vi "Tcp ip main.vi"() -> ()   [LabVIEW 2017]
uses:
  tcp ip server.lvclass
  Q Driver/Controls/IPC-TCP IP-Q driver-Q Options.ctl
  Q Driver/Controls/IPC-TCP IP-Q driver-En Q Element.ctl
panel:
  in  "error in (no error)":errorcluster
  out "error out":errorcluster
  out "Write Data":dbl
  out "Read Data":dbl
  in  "stop":bool
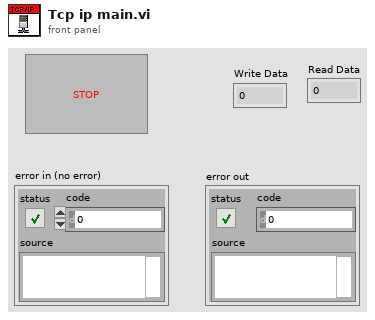
[diagram p1: front panel]
types:
  T1 = typedef "IPC-TCP IP-Q driver-Q Options.ctl" = enum16{"En Q N", "De Q", "Init", "En Q N Stack", "Flush", "Close"}
  T2 = typedef "IPC-TCP IP-Q driver-En Q Element.ctl" = cluster{"State":string, "Data":variant}
  T3 = enum16{"Init", "send", "receive", "Read Received Data", "Write Send Data"}
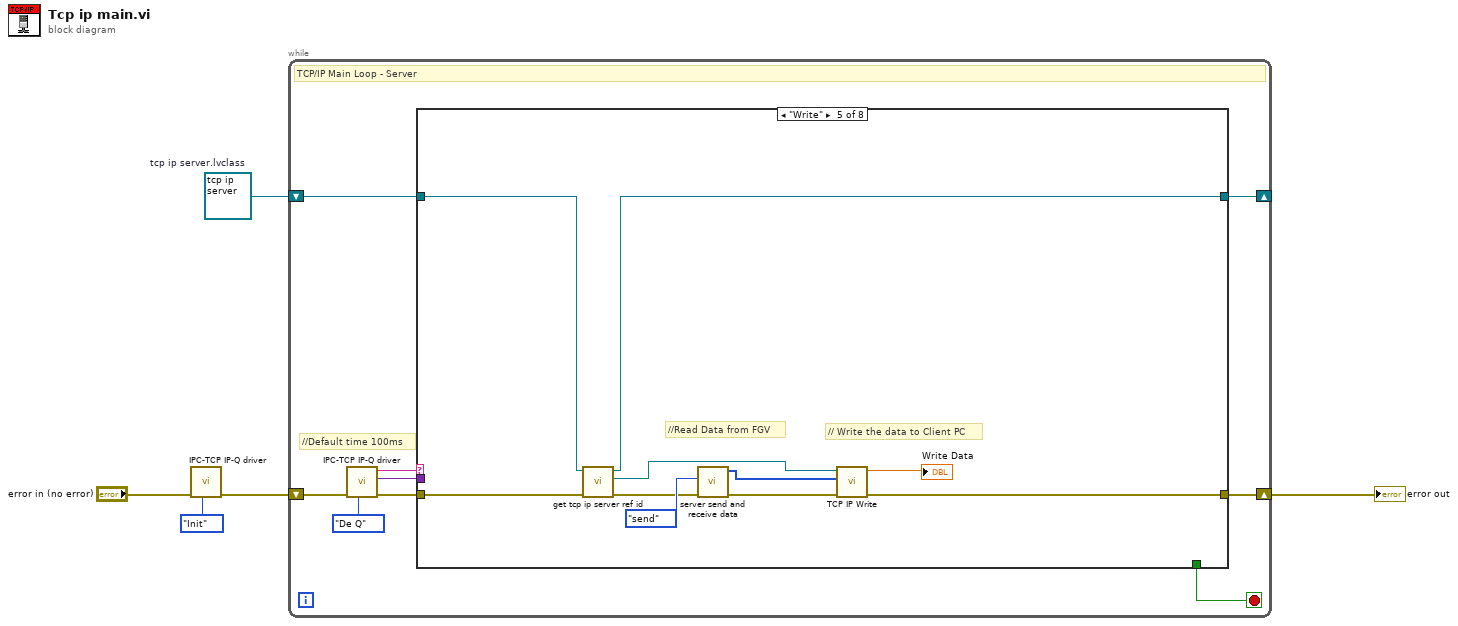
[diagram p0: block diagram]
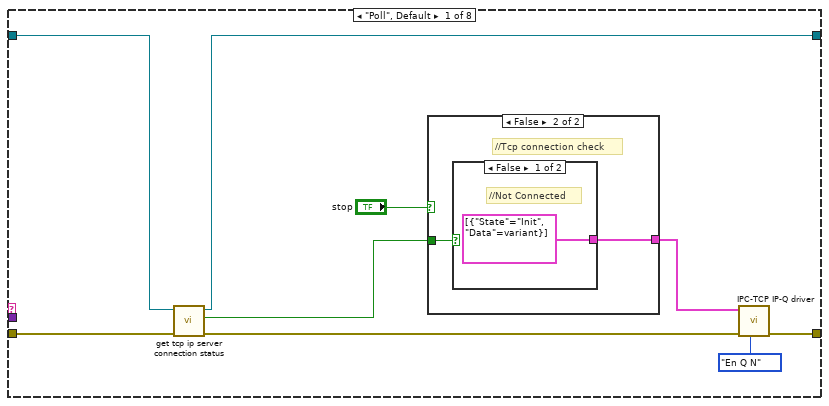
[diagram p2: hidden frame]
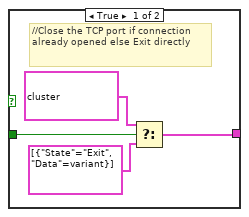
[diagram p3: hidden frame]
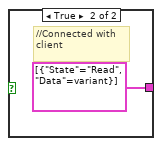
[diagram p4: hidden frame]
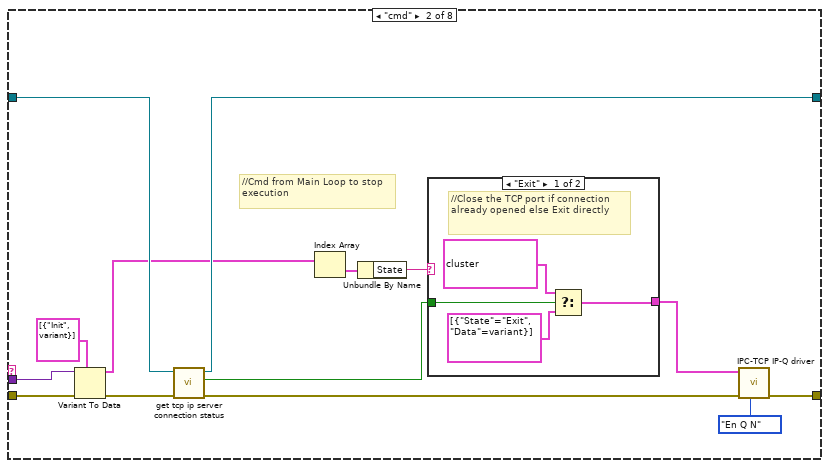
[diagram p5: hidden frame]
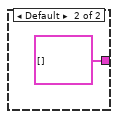
[diagram p6: hidden frame]
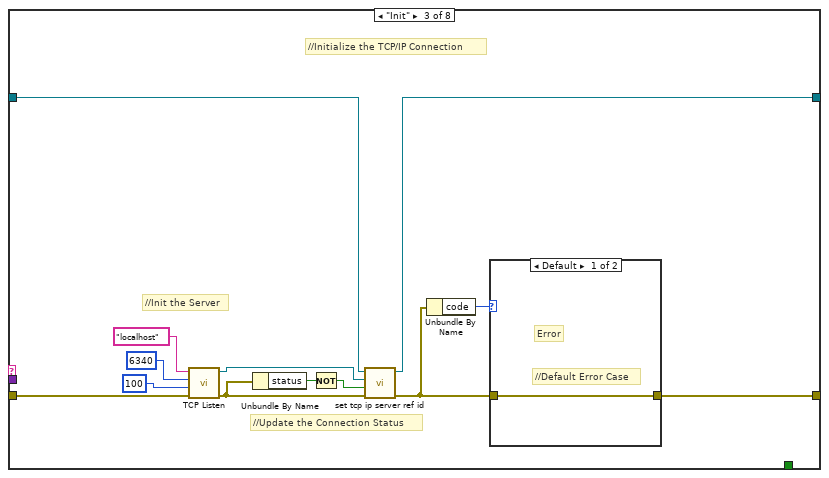
[diagram p7: hidden frame]
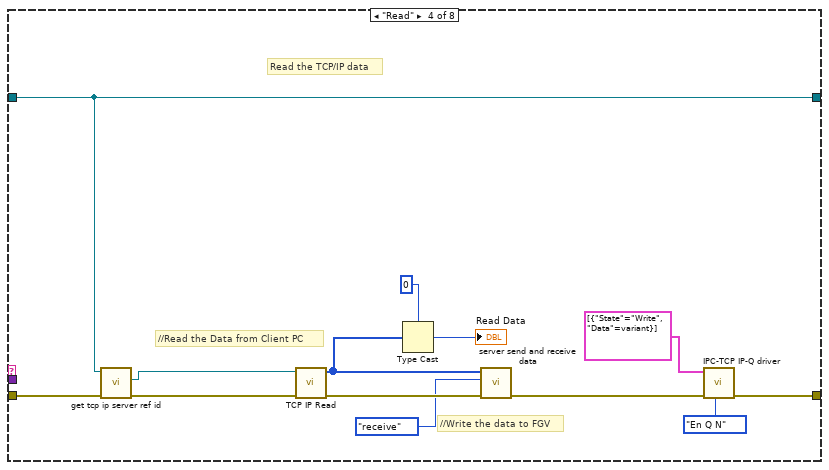
[diagram p9: hidden frame]
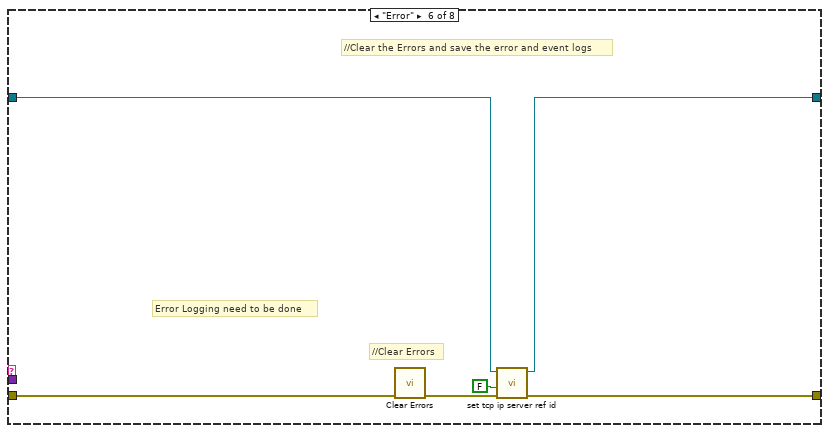
[diagram p10: hidden frame]
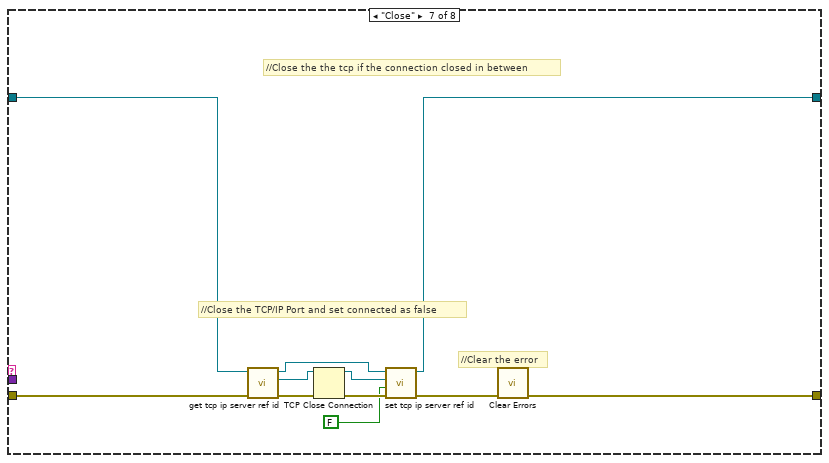
[diagram p11: hidden frame]
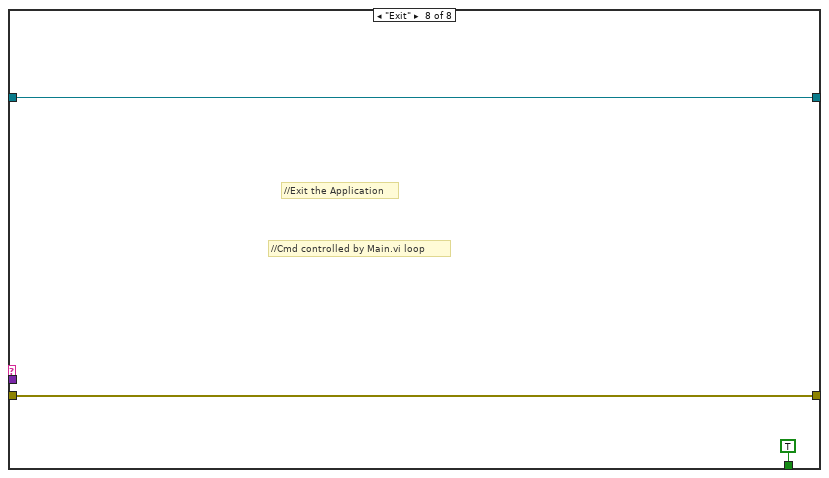
[diagram p12: hidden frame]
diagram:
  w5 = refnum<class "tcp ip server.lvclass"> refnum  # tcp ip server.lvclass
  n1 = call "IPC-TCP IP-Q driver.vi"("Q Options"=IPC-TCP_IP-Q_driver-Q_Options."Init", "error in (no error)"="error in (no error)") -> ("error out"=w4:errorcluster)  [unwired: 7 in, 2 out]
  n2 = while {
    shift-right: [w13] -> _
    shift-left: w5 -> [w14]
    shift-right: [w12] -> w2
    shift-left: w4 -> [w9]
    stop <- w11 stop-if-true
    # "//Default time 100ms"
    # "TCP/IP Main Loop - Server"
    n3 = call "IPC-TCP IP-Q driver.vi"("Q Options"=IPC-TCP_IP-Q_driver-Q_Options."De Q", "error in (no error)"=w9) -> ("error out"=w8:errorcluster, "Data"=w6:variant, "State"=w7:string)  [unwired: 7 in]
    n4 = case shown="\"Write\"" w7 {
      tunnel: w14 -> [w23 w45 w61 w75 w82 w90 w102 w106]
      tunnel: [w22 w44 w60 w75 w78 w89 w97 w106] -> w13
      tunnel: [w19 w41 w54 w67 w80 w88 w94 w105] -> w12
      tunnel: w8 -> [w16 w35 w59 w77 w86 w93 w103 w105]
      tunnel: [_ _ _ _ _ _ _ TRUE ("stop")] -> w11
      tunnel: w6 -> [_ w39 _ _ _ _ _ _]
      frame "Poll", Default {
        n5 = call-dynamic "get tcp ip server connection status.vi"("error in (no error)"=w16, "tcp ip server in"=w23) -> ("error out"=w20:errorcluster, "Connected?"=w18:bool, "tcp ip server out"=w22:refnum<class "tcp ip server.lvclass">)  [unwired: 7 in]
        n6 = case shown="False" "stop" {
          tunnel: w18 -> [w26 w29]
          tunnel: [w25 w28] -> w17
          frame True {
            # "//Close the TCP port if connection already opened else Exit directly"
            n7 = Select(t=T2[] [{"State"="Close", "Data"=variant}, {"State"="Exit", "Data"=variant}] ("En Q"), s=w26, f=T2[] [{"State"="Exit", "Data"=variant}] ("En Q")) -> (s? t:f=w25:T2[])
          }
          frame False {
            # "//Tcp connection check"
            n8 = case shown="False" w29 {
              tunnel: [T2[] [{"State"="Init", "Data"=variant}] ("En Q") T2[] [{"State"="Read", "Data"=variant}] ("En Q")] -> w28
              frame False {
                # "//Not Connected"
              }
              frame True {
                # "//Connected with client"
              }
            }
          }
        }
        n9 = call "IPC-TCP IP-Q driver.vi"("Q Options"=IPC-TCP_IP-Q_driver-Q_Options."En Q N", "error in (no error)"=w20, "En Q"=w17) -> ("error out"=w19:errorcluster)  [unwired: 6 in, 2 out]
      }
      frame "cmd" {
        # "//Cmd from Main Loop to stop execution"
        n10 = Variant To Data(error in=w35, type=T2[] [{"State"="Init", "Data"=variant}] ("En Q"), Variant=w39) -> (data=w36:T2[], error out=w32:errorcluster)
        n11 = call-dynamic "get tcp ip server connection status.vi"("error in (no error)"=w32, "tcp ip server in"=w45) -> ("error out"=w42:errorcluster, "Connected?"=w33:bool, "tcp ip server out"=w44:refnum<class "tcp ip server.lvclass">)  [unwired: 7 in]
        n12 = Index Array(array=w36) -> (element=w38:T2)  [unwired: 1 in]
        n13 = Unbundle By Name(w38) -> ("State"=w34:string)
        n14 = case shown="\"Exit\"" w34 {
          tunnel: w33 -> [w48 _]
          tunnel: [w47 T2[] [] ("En Q")] -> w37
          frame "Exit" {
            # "//Close the TCP port if connection already opened else Exit directly"
            n15 = Select(t=T2[] [{"State"="Close", "Data"=variant}, {"State"="Exit", "Data"=variant}] ("En Q"), s=w48, f=T2[] [{"State"="Exit", "Data"=variant}] ("En Q")) -> (s? t:f=w47:T2[])
          }
          frame Default {
          }
        }
        n16 = call "IPC-TCP IP-Q driver.vi"("Q Options"=IPC-TCP_IP-Q_driver-Q_Options."En Q N", "error in (no error)"=w42, "En Q"=w37) -> ("error out"=w41:errorcluster)  [unwired: 6 in, 2 out]
      }
      frame "Init" {
        # "//Initialize the TCP/IP Connection"
        # "//Update the Connection Status"
        # "//Init the Server"
        n17 = call <vilib>:"TCP Listen.vi"("error in (no error)"=w59, "timeout ms (wait forever: -1)"=100, "port"=u16 6340, "service name"="localhost") -> ("error out"=w53:errorcluster, "connection ID"=w62:refnum<k5>)  [unwired: 3 in, 3 out]
        n18 = Unbundle By Name(w53) -> ("status"=w52:bool)
        n19 = Not(x=w52) -> (.not. x?=w51:bool)
        n20 = call-dynamic "set tcp ip server ref id.vi"("error in (no error)"=w53, "Connected?"=w51, "tcp ID"=w62, "tcp ip server in"=w61) -> ("error out"=w55:errorcluster, "tcp ip server out"=w60:refnum<class "tcp ip server.lvclass">)  [unwired: 6 in]
        n21 = Unbundle By Name(w55) -> ("code"=w56:i32)
        n22 = case shown="Default" w56 {
          tunnel: w55 -> [w64 _]
          tunnel: [w64 _] -> w54
          frame Default {
            # "//Default Error Case"
            # "Error"
          }
          frame 0, 56 {
            # "//Go to Default Case"
            # "Time out"
          }
        }
      }
      frame "Read" {
        # "Read the TCP/IP data"
        # "//Write the data to FGV"
        # "//Read the Data from Client PC"
        n23 = call-dynamic "get tcp ip server ref id.vi"("error in (no error)"=w77, "tcp ip server in"=w75) -> ("error out"=w76:errorcluster, "tcp ID"=w74:refnum<k5>)  [unwired: 7 in, 1 out]
        n24 = call "TCP IP Read.vi"("error in (no error)"=w76, "TCP Network Connection in"=w74) -> ("error out"=w73:errorcluster, "Data Out"=w70:i32[])  [unwired: 8 in]
        n25 = Type Cast(type=0, x=w70) -> (*(type *) &x=→"Read Data":i32)
        n26 = call "server send and receive data .vi"("error in (no error)"=w73, "Option"=T3."receive", "Data in"=w70) -> ("error out"=w65:errorcluster)  [unwired: 7 in, 1 out]
        n27 = call "IPC-TCP IP-Q driver.vi"("Q Options"=IPC-TCP_IP-Q_driver-Q_Options."En Q N", "error in (no error)"=w65, "En Q"=T2[] [{"State"="Write", "Data"=variant}]) -> ("error out"=w67:errorcluster)  [unwired: 6 in, 2 out]
      }
      frame "Write" {
        # "// Write the data to Client PC"
        # "//Read Data from FGV"
        n28 = call-dynamic "get tcp ip server ref id.vi"("error in (no error)"=w86, "tcp ip server in"=w82) -> ("error out"=w84:errorcluster, "tcp ID"=w85:refnum<k5>, "tcp ip server out"=w78:refnum<class "tcp ip server.lvclass">)  [unwired: 7 in]
        n29 = call "server send and receive data .vi"("error in (no error)"=w84, "Option"=T3."send") -> ("error out"=w83:errorcluster, "Data out"=w81:i32[])  [unwired: 8 in]
        n30 = call "TCP IP Write.vi"("error in (no error)"=w83, "Data in"=w81, "TCP Network Connection in"=w85) -> ("error out"=w80:errorcluster, "Write Data"=→"Write Data":dbl)  [unwired: 7 in]
      }
      frame "Error" {
        # "Error Logging need to be done"
        # "//Clear Errors"
        # "//Clear the Errors and save the error and event logs"
        n31 = call <vilib>:"Clear Errors.vi"("error in (no error)"=w93) -> ("error out"=w92:errorcluster)  [unwired: 5 in, 1 out]
        n32 = call-dynamic "set tcp ip server ref id.vi"("error in (no error)"=w92, "Connected?"=FALSE, "tcp ip server in"=w90) -> ("error out"=w88:errorcluster, "tcp ip server out"=w89:refnum<class "tcp ip server.lvclass">)  [unwired: 7 in]
      }
      frame "Close" {
        # "//Close the the tcp if the connection closed in between"
        # "//Clear the error"
        # "//Close the TCP/IP Port and set connected as false"
        n33 = call-dynamic "get tcp ip server ref id.vi"("error in (no error)"=w103, "tcp ip server in"=w102) -> ("error out"=w101:errorcluster, "tcp ID"=w99:refnum<k5>, "tcp ip server out"=w98:refnum<class "tcp ip server.lvclass">)  [unwired: 7 in]
        n34 = TCP Close Connection(connection ID=w99, error in (no error)=w101) -> (connection ID out=w96:refnum<k5>, error out=w100:errorcluster)  [unwired: 1 in]
        n35 = call-dynamic "set tcp ip server ref id.vi"("Connected?"=FALSE, "tcp ID"=w96, "tcp ip server in"=w98) -> ("tcp ip server out"=w97:refnum<class "tcp ip server.lvclass">)  [unwired: 7 in, 1 out]
        n36 = call <vilib>:"Clear Errors.vi"("error in (no error)"=w100) -> ("error out"=w94:errorcluster)  [unwired: 5 in, 1 out]
      }
      frame "Exit" {
        # "//Cmd controlled by Main.vi loop"
        # "//Exit the Application"
      }
    }
  }
  "error out" <- w2
